vi "Read Post.vi"(8 "Error In":errorcluster, 11 "Mock In":refnum<class "Mock Compile Hook.lvclass">) -> (0 "Error Out":errorcluster, 2 "Post":string, 3 "Mock Out":refnum<class "Mock Compile Hook.lvclass">)   [LabVIEW 2018, in "Tests.lvlib" / "Compile.lvlib" / "Mock Compile Hook.lvclass"]
uses:
  Mock Compile Hook.lvclass
  Mock Compile Hook.lvclass/Mock Compile Hook.ctl
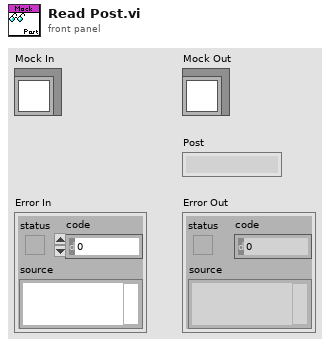
[diagram p1: front panel]
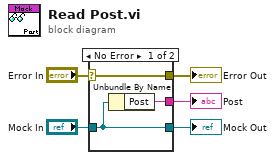
[diagram p0: block diagram]
diagram:
  n1 = case shown="No Error" "Error In" {
    selector: "Error In" -> [w8 w9]
    tunnel: [w8 w9] -> w4
    tunnel: [w7 w10] -> w2
    tunnel: "Mock In" -> [w7 w10]
    tunnel: [w6 _] -> w1
    frame No Error {
      n2 = Unbundle By Name(w7) -> ("Post"=w6:string)
    }
    frame Error {
    }
  }
  "Error Out" <- w4
  "Mock Out" <- w2
  "Post" <- w1
